vi "Localize_Particles-9.vi"(4 "# channel":u8, 5 "[IN] Filtering Settings":T1, 6 "[IN] Destination Image":T2, 7 "error IN":errorcluster, 8 "[IN] Sigma":dbl min=0.1, 9 "Keep Nega-\ntive Values?":bool, 10 "[IN] Frame":T2) -> (0 "error OUT":errorcluster, 2 "[OUT] Histogram Graph":T3 {"Incremental Value" format="%.2f"; "Starting Value" format="%.2f"}, 3 "[OUT] LoG Processed Image":T2)   [LabVIEW 2013]
doc: "Performing the LoG image processing"
uses:
  <vilib>/vision/Image Controls.llb/IMAQ Image.ctl
  <vilib>/vision/NI_Vision_Development_Module.lvlib
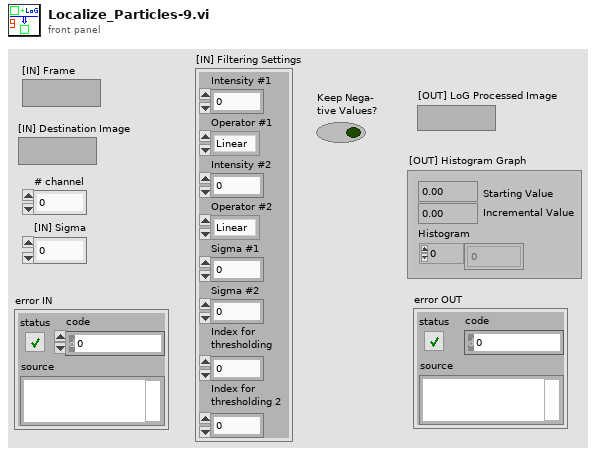
[diagram p1: front panel]
types:
  T1 = cluster{"Intensity #1":sgl, "Operator #1":enum32{"Linear", "Log", "Exp", "Square", "Square root", "Power X", "Power 1/X"}, "Intensity #2":sgl, "Operator #2":enum32{"Linear", "Log", "Exp", "Square", "Square root", "Power X", "Power 1/X"}, "Sigma #1":dbl, "Sigma #2":dbl, "Index for \nthresholding":u8, "Index for \nthresholding 2":u8}
  T2 = typedef "IMAQ Image.ctl" = refnum<image>
  T3 = cluster{"Starting Value":sgl, "Incremental Value":sgl, "Histogram":u32[]}
  T4 = enum32{"Linear", "Log", "Exp", "Square", "Square root", "Power X", "Power 1/X"}
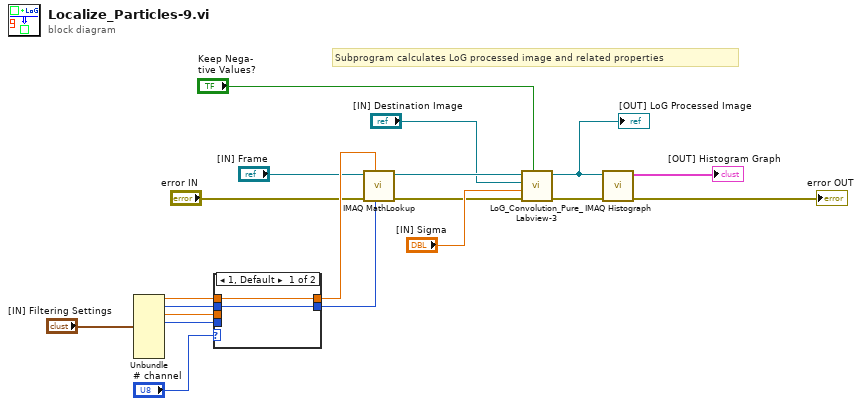
[diagram p0: block diagram]
diagram:
  # "Subprogram calculates LoG processed image and related properties"
  n1 = Unbundle("[IN] Filtering Settings") -> ("Intensity #1"=w17:sgl, "Operator #1"=w16:T4, "Intensity #2"=w13:sgl, "Operator #2"=w12:T4)  [unwired: 4 out]
  n2 = case shown="1, Default" "# channel" {
    tunnel: w17 -> [w21 _]
    tunnel: w16 -> [w20 _]
    tunnel: [w21 w23] -> w15
    tunnel: [w20 w22] -> w14
    tunnel: w13 -> [_ w23]
    tunnel: w12 -> [_ w22]
    frame 1, Default {
    }
    frame 2 {
    }
  }
  n3 = call "IMAQ MathLookup"("Operator"=w14, "X Value"=w15, "error in (no error)"="error IN", "Image Src"="[IN] Frame") -> ("error out"=w5:errorcluster, "Image Dst Out"=w6:T2)  [unwired: 6 in]
  n4 = call "LoG_Convolution_Pure_Labview-3.vi"("Keep Nega-\ntive Values?"="Keep Nega-\ntive Values?", "error IN"=w5, "[IN] Sigma"="[IN] Sigma", "[IN] Processed Image"="[IN] Destination Image", "[IN] Source Image"=w6) -> ("error out"=w2:errorcluster, "[OUT] Processed Image"=w1:T2)  [unwired: 2 in]
  "[OUT] LoG Processed Image" <- w1
  n5 = call "IMAQ Histograph"("error in (no error)"=w2, "Image"=w1) -> ("error out"=→"error OUT":errorcluster, "Histogram Graph"=→"[OUT] Histogram Graph":T3)  [unwired: 6 in, 2 out]
